vi "Main.vi"() -> ()   [LabVIEW 2017]
uses:
  <vilib>/Analysis/baseanly.llb/Mean (DBL).vi
  SmartMotor_class/SmartMotor.lvclass
  <vilib>/Analysis/NI_AALBase.lvlib
panel:
  out "Moving Average":dbl
  in  "Move Motor CCW":bool
  out "Motor Aboslute Position":i32(graph)
  out "Motor Abosolute Position":i32
  out "Motor Torque":T1(graph)
  out "Motor Torque (Filtered)":dbl format="%#.0f"
  in  "Stop Motor":bool
  in  "Move Motor CW":bool
  in  "Quit Program":bool
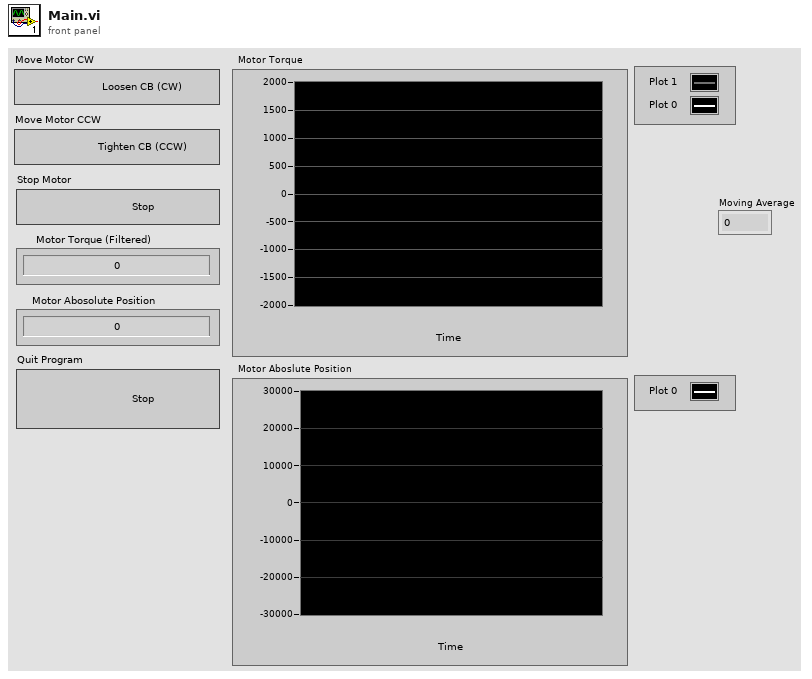
[diagram p1: front panel]
types:
  T1 = cluster{"Motor Torque":i32, "Moving Average":dbl}
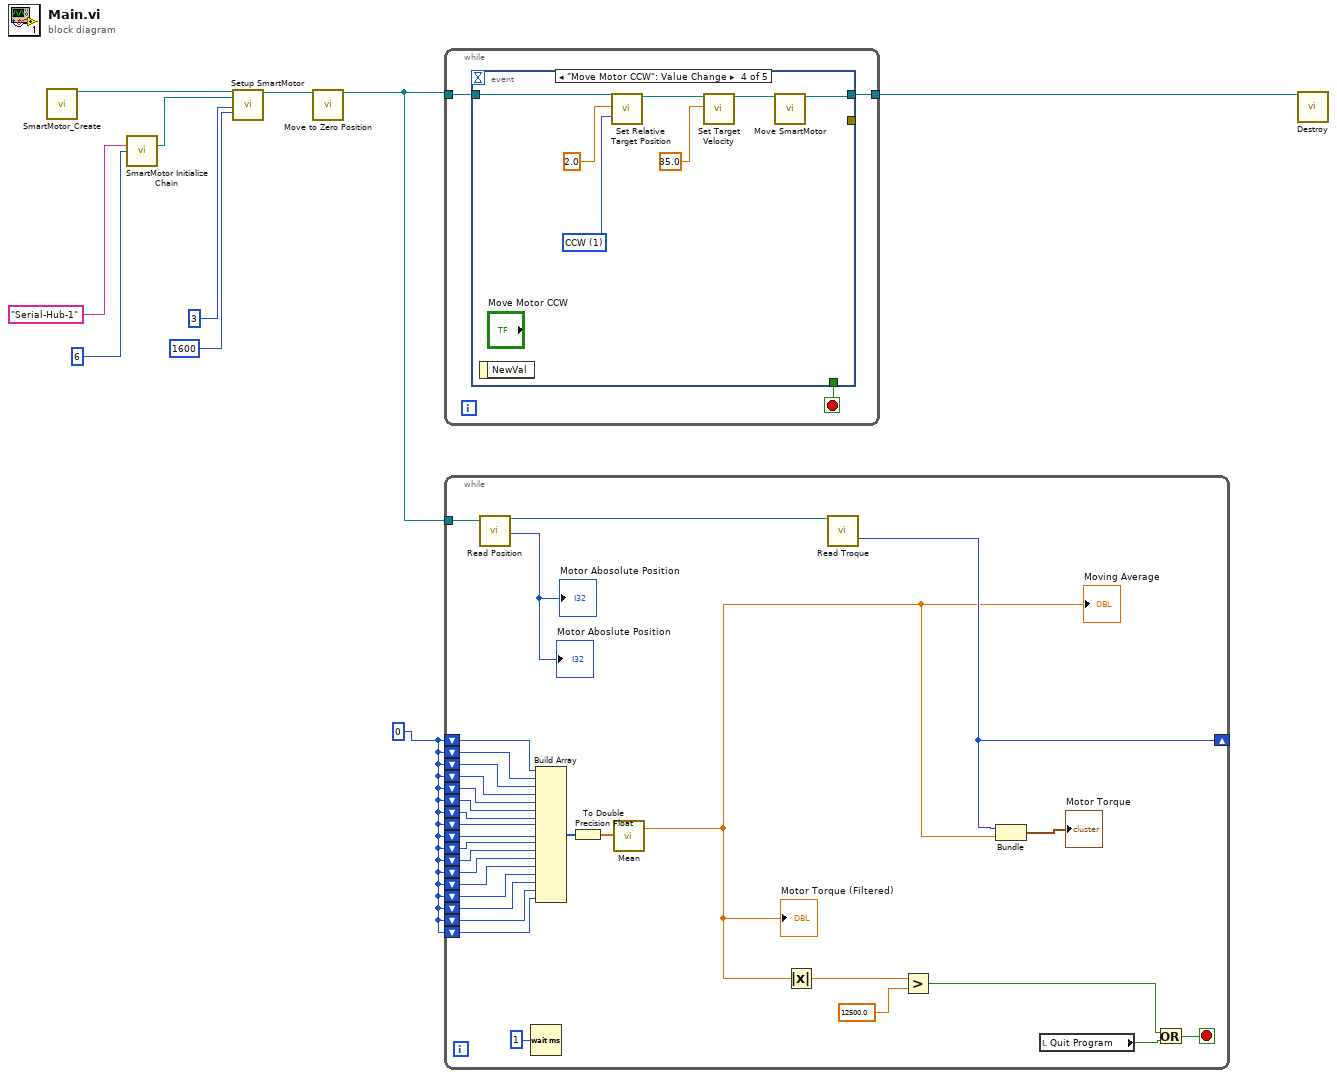
[diagram p0: block diagram]
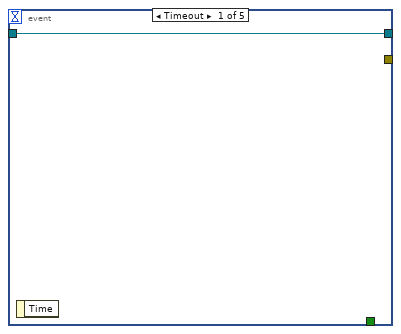
[diagram p2: hidden frame]
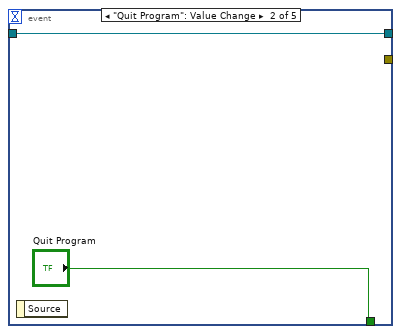
[diagram p3: hidden frame]
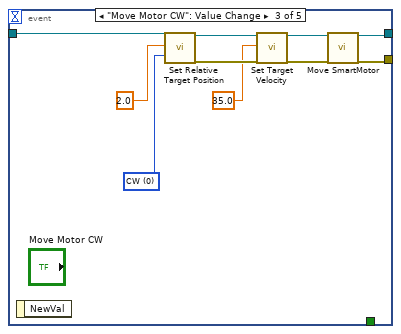
[diagram p4: hidden frame]
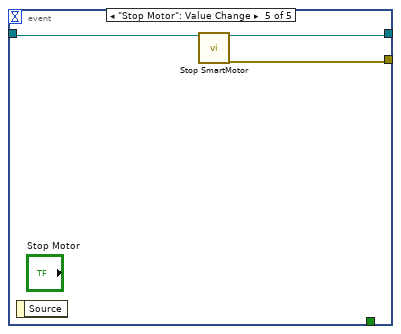
[diagram p5: hidden frame]
diagram:
  w7 = 0
  n1 = call "SmartMotor_Create.vi"() -> ("reference out"=w6:refnum<class "SmartMotor.lvclass">)  [unwired: 18 in, 1 out]
  n2 = call "SmartMotor Initialize Chain.vi"("SmartMotor Chain VISA Resource"="Serial-Hub-1" ("Computer COM Port Name (Allias)"), "Number of Motors In Motor Chain"=6) -> ("SmartMotor Chain VISA Session"=w1:refnum<visa-resource-name>)  [unwired: 11 in, 2 out]
  n3 = call-dynamic "Setup SmartMotor.vi"("reference in"=w6, "SmartMotor Chain VISA Session"=w1, "SmartMotor Chain Address"=3, "Screwdriver Torque Limit"=1600) -> ("reference out"=w10:refnum<class "SmartMotor.lvclass">)  [unwired: 13 in, 2 out]
  n4 = call-dynamic "Move to Zero Position.vi"("reference in"=w10) -> ("reference out"=w8:refnum<class "SmartMotor.lvclass">)  [unwired: 17 in, 1 out]
  n5 = while {
    tunnel: w8 -> [w12]
    tunnel: [w11] -> w9
    stop <- w13 stop-if-true
    n6 = event shown="[3] \"Move Motor CCW\": Value Change" {
      selector: _ -> [_ _ _ _ _]
      dyn-events: _ -> [_ _ _ _ _]
      timeout: _ -> [_ _ _ _ _]
      tunnel: [_ "Quit Program" _ _ _] -> w13
      tunnel: w12 -> [w14 w16 w26 w29 w35]
      tunnel: [w14 w16 w17 w27 w36] -> w11
      tunnel: [_ _ w19 _ w34] -> _
      event Timeout {
        n7 = event-data() -> ()  [unwired: 1 in, 1 out]
      }
      event "Quit Program": Value Change {
        n8 = event-data() -> ()  [unwired: 1 in, 1 out]
      }
      event "Move Motor CW": Value Change {
        w21 = u16 0 items=["CW", "CCW"] ("Rotation Direction")
        n9 = event-data() -> ()  [unwired: 1 in, 1 out]
        n10 = call-dynamic "Set Relative Target Position.vi"("reference in"=w26, "Relative Target Position (Revolutions)"=2.0, "Rotation Direction"=w21) -> ("reference out"=w25:refnum<class "SmartMotor.lvclass">, "error out"=w24:errorcluster)  [unwired: 15 in]
        n11 = call-dynamic "Set Target Velocity.vi"("reference in"=w25, "Target Velocity (RPM)"=35.0, "error in (no error)"=w24) -> ("reference out"=w18:refnum<class "SmartMotor.lvclass">, "error out"=w23:errorcluster)  [unwired: 15 in]
        n12 = call-dynamic "Move SmartMotor.vi"("reference in"=w18, "error in (no error)"=w23) -> ("reference out"=w17:refnum<class "SmartMotor.lvclass">, "error out"=w19:errorcluster)  [unwired: 16 in]
      }
      event "Move Motor CCW": Value Change {
        w31 = u16 1 items=["CW", "CCW"] ("Rotation Direction")
        n13 = event-data() -> ()  [unwired: 1 in, 1 out]
        n14 = call-dynamic "Set Relative Target Position.vi"("reference in"=w29, "Relative Target Position (Revolutions)"=2.0, "Rotation Direction"=w31) -> ("reference out"=w33:refnum<class "SmartMotor.lvclass">)  [unwired: 15 in, 1 out]
        n15 = call-dynamic "Set Target Velocity.vi"("reference in"=w33, "Target Velocity (RPM)"=35.0) -> ("reference out"=w28:refnum<class "SmartMotor.lvclass">)  [unwired: 16 in, 1 out]
        n16 = call-dynamic "Move SmartMotor.vi"("reference in"=w28) -> ("reference out"=w27:refnum<class "SmartMotor.lvclass">)  [unwired: 17 in, 1 out]
      }
      event "Stop Motor": Value Change {
        n17 = event-data() -> ()  [unwired: 1 in, 1 out]
        n18 = call-dynamic "Stop SmartMotor.vi"("reference in"=w35) -> ("reference out"=w36:refnum<class "SmartMotor.lvclass">, "error out"=w34:errorcluster)  [unwired: 17 in]
      }
    }
  }
  n19 = while {
    tunnel: w8 -> [w62]
    shift-right: [w38] -> _
    shift-left: w7 -> [w59]
    shift-left: w7 -> [w58]
    shift-left: w7 -> [w57]
    shift-left: w7 -> [w54]
    shift-left: w7 -> [w53]
    shift-left: w7 -> [w52]
    shift-left: w7 -> [w51]
    shift-left: w7 -> [w50]
    shift-left: w7 -> [w49]
    shift-left: w7 -> [w48]
    shift-left: w7 -> [w47]
    shift-left: w7 -> [w46]
    shift-left: w7 -> [w45]
    shift-left: w7 -> [w44]
    shift-left: w7 -> [w43]
    shift-left: w7 -> [w42]
    shift-left: w7 -> [w41]
    stop <- w63 stop-if-true
    n20 = call-dynamic "Read Position.vi"("reference in"=w62) -> ("reference out"=w61:refnum<class "SmartMotor.lvclass">, "Motor Absolute Position"=→"Motor Abosolute Position" →"Motor Aboslute Position":i32)  [unwired: 15 in, 2 out]
    n21 = Wait (ms)(milliseconds to wait=u32 1) -> ()  [unwired: 1 out]
    n22 = Build Array(w59, w58, w57, w54, w53, w52, w51, w50, w49, w48, w47, w46, w45, w44, w43, w42, w41) -> (w56:i32[])
    n23 = To Double Precision Float(number=w56) -> (double precision float=w55:dbl[])
    n24 = call-poly <vilib>:"Mean.vi"("X"=w55) -> ("mean"=w37:dbl)  [unwired: 1 out]
    "Motor Torque (Filtered)" <- w37
    "Moving Average" <- w37
    n25 = Absolute Value(x=w37) -> (abs(x)=w40:dbl)
    n26 = call-dynamic "Read Troque.vi"("reference in"=w61) -> ("Motor Torque"=w38:i32)  [unwired: 16 in, 2 out]
    n27 = Greater?(x=w40, y=12500.0) -> (0:w65:bool)
    n28 = Bundle("Motor Torque"=w38, "mean"=w37) -> (→"Motor Torque":cluster{"Motor Torque":i32, "mean":dbl})  [unwired: 1 in]
    n29 = local read "Quit Program"() -> (w64:bool)
    n30 = Or(x=w65, y=w64) -> (x .or. y?=w63:bool)
  }
  n31 = call-dynamic "Destroy.vi"("reference in"=w9) -> ()  [unwired: 17 in, 2 out]
